vi "PH_SSAC.Frame2Rectangle.vi"(1 "Frame":cluster{"x":u32, "dx":u32, "y":u32, "dy":u32}) -> (0 "Rectangle":T1)   [LabVIEW 2014, in "PH_SSAC.lvlib"]
doc: "This VI converts Frames as used in this class to a rectangle as used in vision VIs."
uses:
  PH_SSAC.lvlib
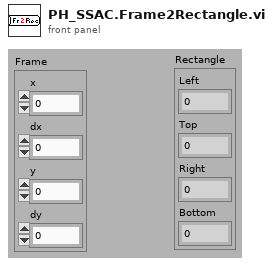
[diagram p1: front panel]
types:
  T1 = cluster{"Left":i32, "Top":i32, "Right":i32, "Bottom":i32}
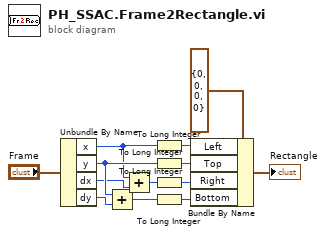
[diagram p0: block diagram]
diagram:
  n1 = Unbundle By Name("Frame") -> ("x"=w6:u32, "y"=w9:u32, "dx"=w5:u32, "dy"=w8:u32)
  n2 = Add(x=w9, y=w8) -> (x+y=w7:u32)
  n3 = Add(x=w6, y=w5) -> (x+y=w4:u32)
  n4 = To Long Integer(number=w6) -> (32bit integer=w13:i32)
  n5 = To Long Integer(number=w9) -> (32bit integer=w12:i32)
  n6 = To Long Integer(number=w4) -> (32bit integer=w11:i32)
  n7 = To Long Integer(number=w7) -> (32bit integer=w10:i32)
  n8 = Bundle By Name(cluster=T1 {"Left"=0, "Top"=0, "Right"=0, "Bottom"=0} ("Rectangle"), "Left"=w13, "Top"=w12, "Right"=w11, "Bottom"=w10) -> (→"Rectangle":T1)
